vi "LED_Execute.vi"   [LabVIEW 2018]
uses:
  <vilib>/Rock Robotics/WPI/ThirdParty/Phoenix-LabVIEW/CANifier/CTRE_CANifier_LEDChannel.ctl
  Global_Variables/LED_Globals.vi
  Global_Variables/Sensor_Values.vi
types:
  T1 = typedef "CTRE_CANifier_DeviceRef.ctl" = cluster{"DeviceStatus":errorcluster, "Device Number":u8, "Handle":u64, "UsageFrame":u32, "Library Path":path}
  T2 = typedef "CTRE_CANifier_LEDChannel.ctl" = enum32{"LEDChannelA", "LEDChannelB", "LEDChannelC"}
  T3 = cluster{"offsetAngle H":dbl, "offsetAngle V":dbl, "area":dbl, "skew":dbl}
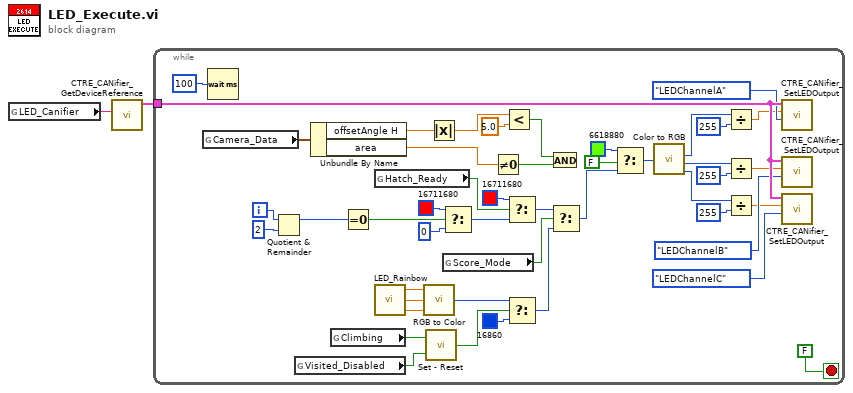
[diagram p0: block diagram]
diagram:
  n1 = global read "LED_Globals.vi" "LED_Canifier"() -> (w2:string)
  n2 = call <vilib>:"CTRE_CANifier_GetDeviceReference.vi"("refnum name"=w2) -> ("CANifierDevRef"=w1:T1)  [unwired: 9 in, 1 out]
  n3 = while {
    tunnel: w1 -> [w46]
    i -> [w39]
    stop <- FALSE stop-if-true
    n4 = global read "Sensor_Values.vi" "Camera_Data"() -> (w10:T3)
    n5 = Wait (ms)(milliseconds to wait=u32 100) -> ()  [unwired: 1 out]
    n6 = Quotient & Remainder(x=w39, y=2) -> (x-y*floor(x/y)=w37:i32)  [unwired: 1 out]
    n7 = global read "LED_Globals.vi" "Visited_Disabled"() -> (w12:bool)
    n8 = Unbundle By Name(w10) -> ("offsetAngle H"=w9:dbl, "area"=w5:dbl)
    n9 = global read "LED_Globals.vi" "Climbing"() -> (w14:bool)
    n10 = Equal To 0?(x=w37) -> (x = 0?=w20:bool)
    n11 = global read "LED_Globals.vi" "Hatch_Ready"() -> (w17:bool)
    n12 = call "LED_Rainbow.vi"() -> ("B"=w41:dbl, "G"=w42:dbl, "R"=w43:dbl)
    n13 = call <vilib>:"RGB to Color.vi"("B"=w41, "G"=w42, "R"=w43) -> ("Color"=w44:u32)
    n14 = call "Set - Reset.vi"("Reset"=w12, "Set"=w14) -> ("Output"=w13:bool)
    n15 = Absolute Value(x=w9) -> (abs(x)=w8:dbl)
    n16 = Select(t=u32 16711680 ("Color"), s=w20, f=u32 0) -> (s? t:f=w16:u32)
    n17 = global read "LED_Globals.vi" "Score_Mode"() -> (w11:bool)
    n18 = Not Equal To 0?(x=w5) -> (x != 0?=w4:bool)
    n19 = Less?(x=w8, y=5.0) -> (x < y?=w6:bool)
    n20 = Select(t=u32 16711680 ("Color"), s=w17, f=w16) -> (s? t:f=w36:u32)
    n21 = Select(t=w44, s=w13, f=u32 16860 ("Color")) -> (s? t:f=w40:u32)
    n22 = And(x=w6, y=w4) -> ()  [unwired: 1 out]
    n23 = Select(t=w36, s=w11, f=w40) -> (s? t:f=w23:u32)
    n24 = Select(t=u32 6618880 ("Color"), s=FALSE, f=w23) -> (s? t:f=w22:u32)
    n25 = call <vilib>:"Color to RGB.vi"("Color"=w22) -> ("R"=w32:u8, "G"=w31:u8, "B"=w30:u8)  [unwired: 1 out]
    n26 = Divide(x=w32, y=u8 255) -> (x/y=w26:dbl)
    n27 = Divide(x=w31, y=u8 255) -> (x/y=w25:dbl)
    n28 = Divide(x=w30, y=u8 255) -> (x/y=w24:dbl)
    n29 = call <vilib>:"CTRE_CANifier_SetLEDOutput.vi"("LEDChannel"=CTRE_CANifier_LEDChannel."LEDChannelA", "Percent Output"=w26, "CANifierDevRef"=w46) -> ()  [unwired: 7 in, 2 out]
    n30 = call <vilib>:"CTRE_CANifier_SetLEDOutput.vi"("LEDChannel"=CTRE_CANifier_LEDChannel."LEDChannelB", "Percent Output"=w25, "CANifierDevRef"=w46) -> ()  [unwired: 7 in, 2 out]
    n31 = call <vilib>:"CTRE_CANifier_SetLEDOutput.vi"("LEDChannel"=CTRE_CANifier_LEDChannel."LEDChannelC", "Percent Output"=w24, "CANifierDevRef"=w46) -> ()  [unwired: 7 in, 2 out]
  }
